vi "Notify to MS teams from config.vi"(7 "additional label":string, 8 "working directory":path, 10 "message":string, 11 "title":string) -> ()   [LabVIEW 2022 SP3]
uses:
  <vilib>/Utility/error.llb/Trim Whitespace One-Sided.vi
panel:
  # "cofig file shuld be as follow\n\n```json\n{\n    \"url\": \"some webhook urk\"\n}\n```"
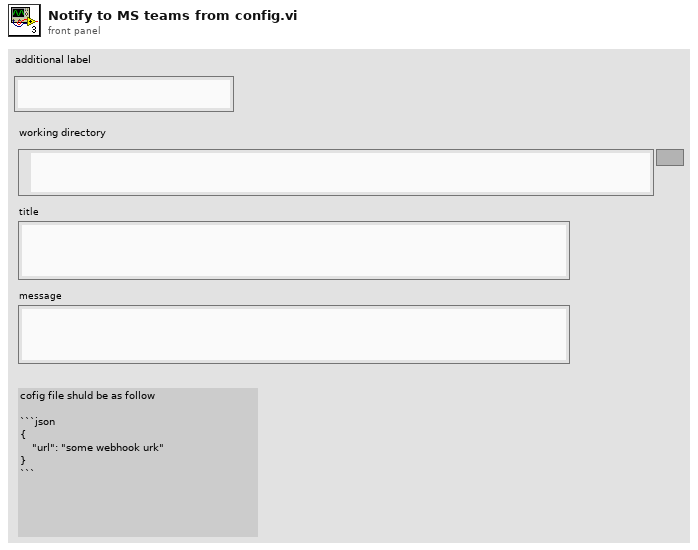
[diagram p1: front panel]
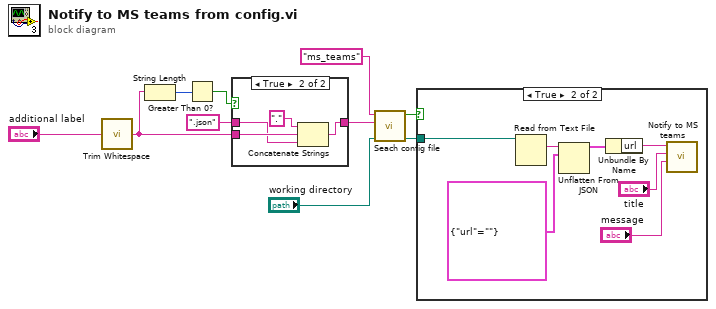
[diagram p0: block diagram]
diagram:
  n1 = call <vilib>:"Trim Whitespace.vi"("string"="additional label") -> ("trimmed string"=w1:string)  [unwired: 1 in]
  n2 = String Length(string=w1) -> (length=w5:i32)
  n3 = Greater Than 0?(x=w5) -> (x > 0?=w4:bool)
  n4 = case shown="True" w4 {
    tunnel: ".json" ("extention") -> [w11 w14]
    tunnel: [w11 w12] -> w2
    tunnel: w1 -> [_ w15]
    frame False {
    }
    frame True {
      n5 = Concatenate Strings("." ("string"), w15, w14) -> (w12:string)
    }
  }
  n6 = call "Seach config file.vi"("working directory"="working directory", "extention"=w2, "pkg name"="ms_teams") -> ("config file path"=w7:path, "config file found?"=w8:bool)  [unwired: 5 in]
  n7 = case shown="True" w8 {
    tunnel: w7 -> [_ w22]
    frame False {
    }
    frame True {
      n8 = Read from Text File(file (use dialog)=w22) -> (text=w21:string)  [unwired: 3 in, 3 out]
      n9 = Unflatten From JSON(JSON string=w21, type and defaults=cluster{"url":string} {"url"=""}) -> (value=w19:cluster{"url":string})  [unwired: 5 in, 1 out]
      n10 = Unbundle By Name(w19) -> ("url"=w18:string)
      n11 = call "Notify to MS teams.vi"("message"="message", "title"="title", "URL"=w18) -> ()  [unwired: 9 in]
    }
  }
